vi "1 Tap 24-Bit RGB.vi"() -> (0 "PixelData":u32)   [LabVIEW 2012]
uses:
  <vilib>/rvi/eio/common/nirviEmuTemplateMethod_errors.vi
  <vilib>/eio/EIONode/EIONode.xnode
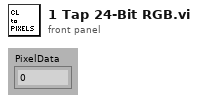
[diagram p1: front panel]
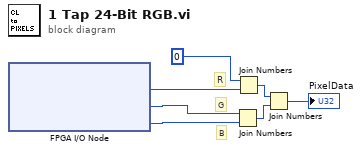
[diagram p0: block diagram]
diagram:
  # "B"
  # "G"
  # "R"
  n1 = xnode "FPGA I/O Node"() -> ("IO Module\\CL Port A"=w5:u8, "IO Module\\CL Port B"=w6:u8, "IO Module\\CL Port C"=w7:u8)  [unwired: 3 in, 3 out]
  n2 = Join Numbers(hi=w6, lo=w7) -> ((hi.lo)=w3:u16)
  n3 = Join Numbers(hi=u8 0, lo=w5) -> ((hi.lo)=w2:u16)
  n4 = Join Numbers(hi=w2, lo=w3) -> ((hi.lo)=→"PixelData":u32)
